vi "GetParam.vi"(8 "error in":errorcluster, 10 "Param":string, 11 "Node ROS":T1={"topic port"=0, "Node"="", "topic"="", "type"="", "node port"=0, "error "={"status"=FALSE, "code"=0, "source"=""}, "Direction"=enum."Node", "APIs"=[], "Update (ms)"=1, "write queue"=1}) -> (0 "error out":errorcluster, 2 "XML Received":string, 3 "Node ROS Out":T1={"topic port"=0, "Node"="", "topic"="", "type"="", "node port"=0, "error "={"status"=FALSE, "code"=0, "source"=""}, "Direction"=enum."Node", "APIs"=[], "Update (ms)"=1, "write queue"=1})   [LabVIEW 2012]
doc: "Reads a parameter from the parameter server. The parameter server must be running at the same address as the ROS master."
uses:
  <userlib>/ROSforLV/ROS/Code/SubVIs/_ROSControl.ctl
  <userlib>/ROSforLV/ROS/Code/SubVIs/_ROSDirection.ctl
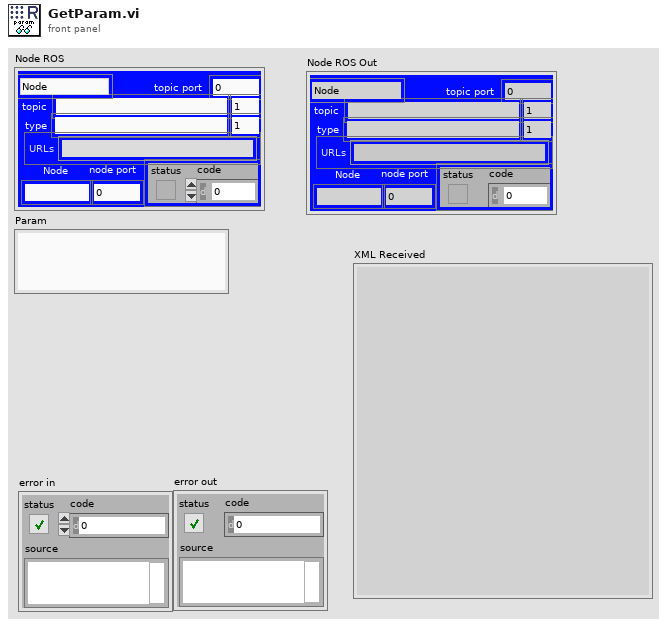
[diagram p1: front panel]
types:
  T1 = typedef "_ROSControl.ctl" = cluster{"topic port":u16, "Node":string, "topic":string, "type":string, "node port":u32, "error ":errorcluster, "Direction":T2, "APIs":string[], "Update (ms)":u16, "write queue":u16}
  T2 = typedef "_ROSDirection.ctl" = enum16{"Node", "Publisher", "Subscriber", "Service Client"}
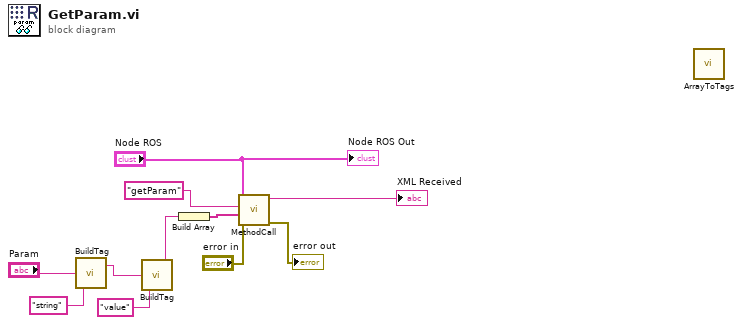
[diagram p0: block diagram]
diagram:
  n1 = call <userlib>:"BuildTag.vi"("tag"="string", "value"="Param") -> ("string out"=w9:string)  [unwired: 2 in]
  n2 = call <userlib>:"BuildTag.vi"("tag"="value", "value"=w9) -> ("string out"=w5:string)  [unwired: 2 in]
  n3 = Build Array(w5) -> (w6:string[])
  n4 = call <userlib>:"MethodCall.vi"("error in"="error in", "Method Params"=w6, "methodName"="getParam", "Node ROS"="Node ROS") -> ("error out"=→"error out":errorcluster, "XML Received"=→"XML Received":string)  [unwired: 6 in]
  n5 = call <userlib>:"ArrayToTags.vi"() -> ()  [unwired: 1 in, 1 out]
  "Node ROS Out" <- "Node ROS"
